vi "AssembleVelocityStats.vi"(7 "TitlePrefix":string, 10 "DataIn":T1) -> (1 "Plug in titles":string[](array[string]), 3 "StatsArray":dbl[](array[numeric]))   [LabVIEW 2020]
uses:
  <vilib>/Analysis/baseanly.llb/Unimode.vi
  <vilib>/Analysis/NI_AALBase.lvlib
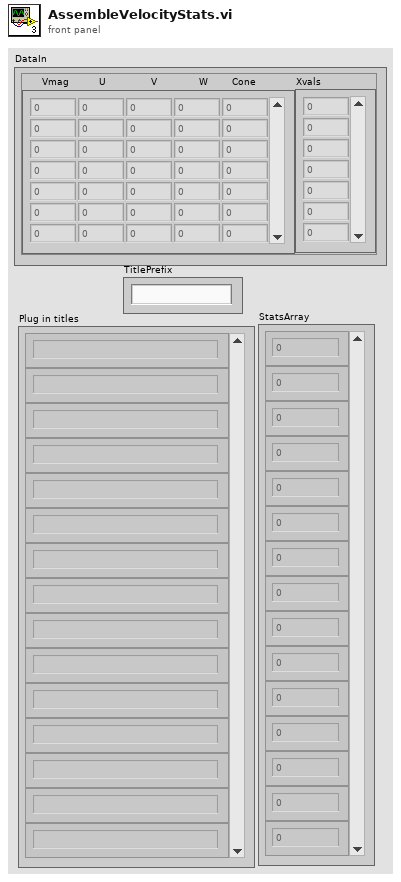
[diagram p1: front panel]
types:
  T1 = cluster{"   Vmag          U               V              W        Cone":dbl[][], "Xvals":i32[]}
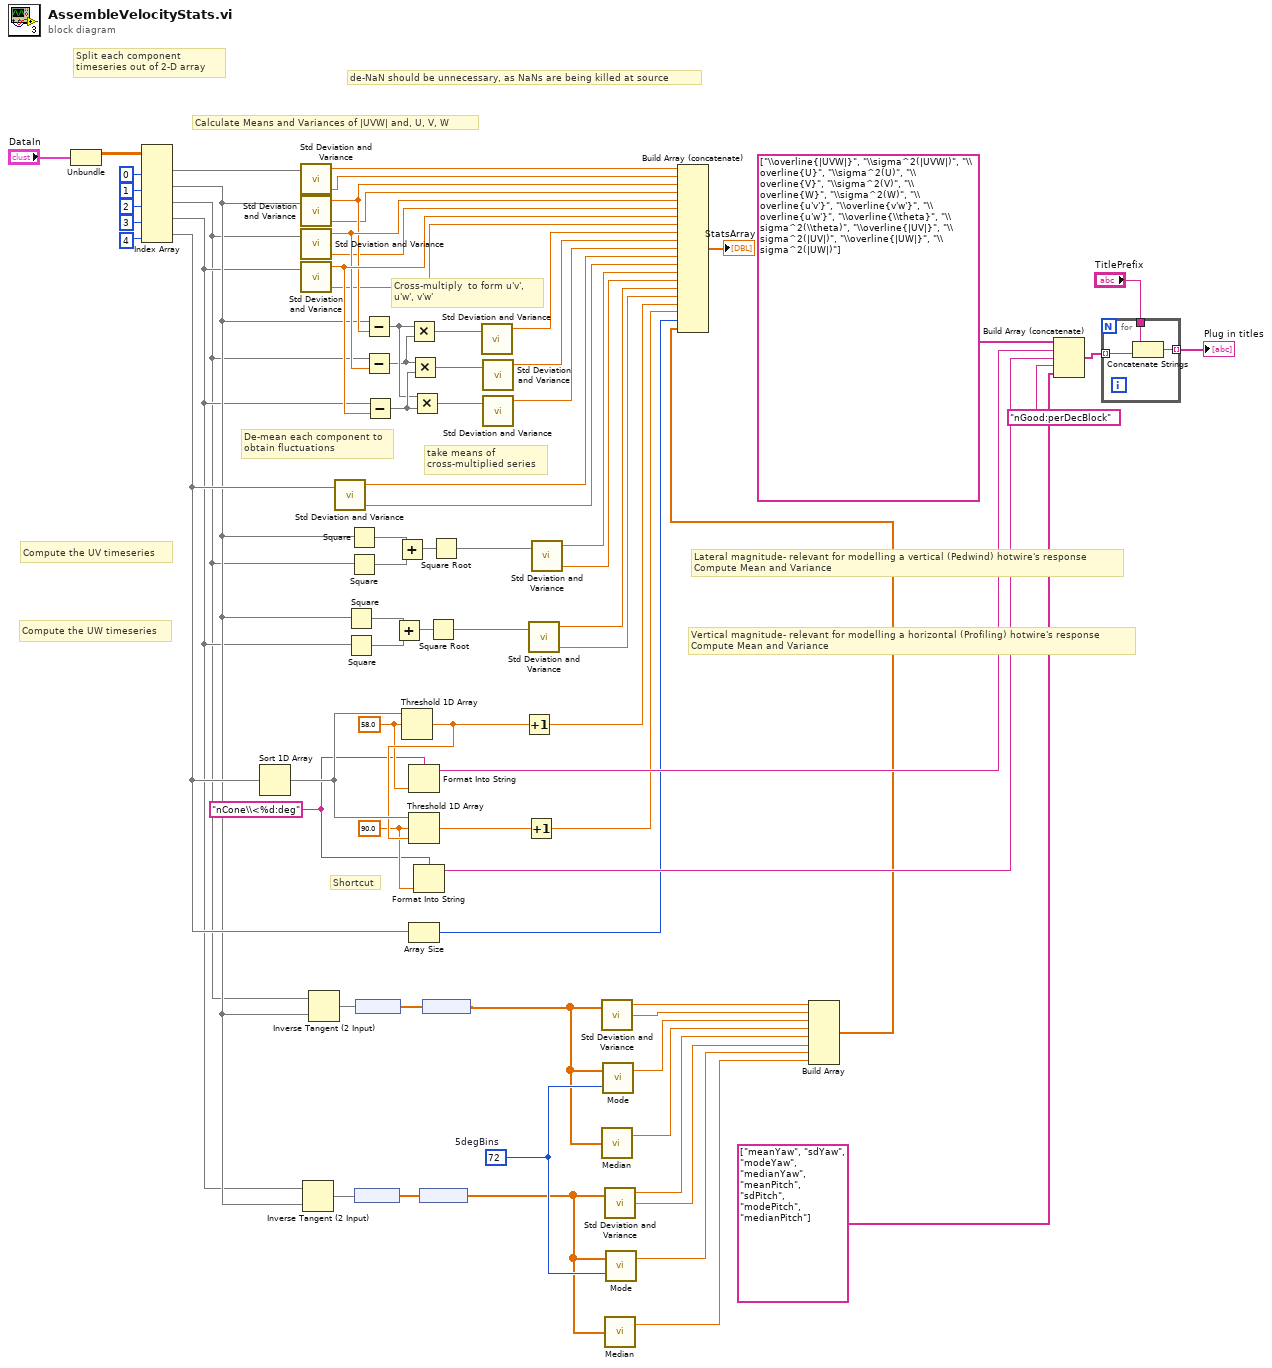
[diagram p0: block diagram]
diagram:
  w13 = 72  # 5degBins
  w31 = "nCone\\<%d:deg" ("format string")
  w32 = 90.0 ("threshold y")
  w33 = 58.0 ("threshold y")
  # "Split each component timeseries out of 2-D array"
  # "Compute the UW timeseries"
  # "Compute the UV timeseries"
  # "take means of cross-multiplied series"
  # "Cross-multiply  to form u'v', u'w', v'w'"
  # "De-mean each component to obtain fluctuations"
  # "Calculate Means and Variances of |UVW| and, U, V, W"
  # "Shortcut"
  # "de-NaN should be unnecessary, as NaNs are being killed at source"
  # "Vertical magnitude- relevant for modelling a horizontal (Profiling) hotwire's response\nCompute Mean and Variance"
  # "Lateral magnitude- relevant for modelling a vertical (Pedwind) hotwire's response\nCompute Mean and Variance"
  n1 = Unbundle("DataIn") -> ("Vmag          U               V              W        Cone"=w26:dbl[][])  [unwired: 1 out]
  n2 = Index Array(array=w26, index (col) #1=0 ("disabled index (col)"), index (col) #2=1 ("index (col)"), index (col) #3=2 ("index (col)"), index (col) #4=3 ("index (col)"), index (col) #5=4 ("index (col)")) -> (element #1=w25:dbl[], element #2=w20:dbl[], element #3=w18:dbl[], element #4=w19:dbl[], element #5=w37:dbl[])  [unwired: 5 in]
  n3 = Sort 1D Array(array=w37) -> (sorted array=w36:dbl[])
  n4 = call <vilib>:"Std Deviation and Variance.vi"("X"=w25) -> ("mean"=w65:dbl, "variance"=w60:dbl)  [unwired: 1 in, 1 out]
  n5 = call <vilib>:"Std Deviation and Variance.vi"("X"=w20) -> ("mean"=w66:dbl, "variance"=w61:dbl)  [unwired: 1 in, 1 out]
  n6 = call <vilib>:"Std Deviation and Variance.vi"("X"=w18) -> ("mean"=w67:dbl, "variance"=w62:dbl)  [unwired: 1 in, 1 out]
  n7 = call <vilib>:"Std Deviation and Variance.vi"("X"=w19) -> ("mean"=w68:dbl, "variance"=w63:dbl)  [unwired: 1 in, 1 out]
  n8 = Inverse Tangent (2 Input)(1:w20, 2:w19) -> (0:w15:dbl[])
  n9 = Inverse Tangent (2 Input)(1:w20, 2:w18) -> (0:w14:dbl[])
  n10 = call <vilib>:"Std Deviation and Variance.vi"("X"=w37) -> ("mean"=w76:dbl, "variance"=w77:dbl)  [unwired: 1 in, 1 out]
  n11 = Square(x=w20) -> (x^2=w40:dbl[])
  n12 = Square(x=w19) -> (x^2=w41:dbl[])
  n13 = Square(x=w20) -> (x^2=w49:dbl[])
  n14 = Square(x=w18) -> (x^2=w48:dbl[])
  n15 = node(w15) -> (w16:dbl[unit][])
  n16 = node(w14) -> (w17:dbl[unit][])
  n17 = Subtract(x=w20, y=w66) -> (x-y=w70:dbl[])
  n18 = Subtract(x=w18, y=w67) -> (x-y=w69:dbl[])
  n19 = Subtract(x=w19, y=w68) -> (x-y=w71:dbl[])
  n20 = Add(x=w40, y=w41) -> (x+y=w42:dbl[])
  n21 = Add(x=w49, y=w48) -> (x+y=w47:dbl[])
  n22 = Threshold 1D Array(2:w33, 3:w36) -> (0:w35:dbl)  [unwired: 1 in]
  n23 = Multiply(x=w70, y=w69) -> (x*y=w52:dbl[])
  n24 = Format Into String(format string=w31, w33) -> (resulting string=w29:string)  [unwired: 2 in, 1 out]
  n25 = Threshold 1D Array(1:w35, 2:w32, 3:w36) -> (0:w34:dbl)
  n26 = Array Size(array=w37) -> (size(s)=w23:i32)
  n27 = Multiply(x=w69, y=w71) -> (x*y=w51:dbl[])
  n28 = Multiply(x=w70, y=w71) -> (x*y=w50:dbl[])
  n29 = Format Into String(format string=w31, w32) -> (resulting string=w28:string)  [unwired: 2 in, 1 out]
  n30 = node(w16) -> (w11:dbl[])
  n31 = node(w17) -> (w12:dbl[])
  n32 = Square Root(x=w42) -> (sqrt(x)=w43:dbl[])
  n33 = Square Root(x=w47) -> (sqrt(x)=w46:dbl[])
  n34 = call <vilib>:"Std Deviation and Variance.vi"("X"=w52) -> ("mean"=w72:dbl)  [unwired: 1 in, 2 out]
  n35 = call <vilib>:"Std Deviation and Variance.vi"("X"=w51) -> ("mean"=w73:dbl)  [unwired: 1 in, 2 out]
  n36 = call <vilib>:"Std Deviation and Variance.vi"("X"=w50) -> ("mean"=w74:dbl)  [unwired: 1 in, 2 out]
  n37 = Increment(x=w35) -> (x+1=w22:dbl)
  n38 = Increment(x=w34) -> (x+1=w21:dbl)
  n39 = call <vilib>:"Std Deviation and Variance.vi"("X"=w43) -> ("mean"=w39:dbl, "variance"=w38:dbl)  [unwired: 1 in, 1 out]
  n40 = call <vilib>:"Std Deviation and Variance.vi"("X"=w46) -> ("mean"=w45:dbl, "variance"=w44:dbl)  [unwired: 1 in, 1 out]
  n41 = call <vilib>:"Std Deviation and Variance.vi"("X"=w12) -> ("mean"=w10:dbl, "standard deviation"=w9:dbl)  [unwired: 1 in, 1 out]
  n42 = call <vilib>:"Median.vi"("X"=w12) -> ("median"=w7:dbl)  [unwired: 1 out]
  n43 = call-poly <vilib>:"Mode.vi"("intervals"=w13, "X"=w12) -> ("mode"=w8:dbl)  [unwired: 1 out]
  n44 = call <vilib>:"Std Deviation and Variance.vi"("X"=w11) -> ("mean"=w6:dbl, "standard deviation"=w5:dbl)  [unwired: 1 in, 1 out]
  n45 = call <vilib>:"Median.vi"("X"=w11) -> ("median"=w3:dbl)  [unwired: 1 out]
  n46 = call-poly <vilib>:"Mode.vi"("intervals"=w13, "X"=w11) -> ("mode"=w4:dbl)  [unwired: 1 out]
  n47 = Build Array(w10, w9, w8, w7, w6, w5, w4, w3) -> (w2:dbl[])
  n48 = Build Array (concatenate)(w65, w60, w66, w61, w67, w62, w68, w63, w72, w73, w74, w76, w77, w45, w44, w39, w38, w22, w21, w23, w2) -> (→"StatsArray":dbl[])
  n49 = Build Array (concatenate)(string[] ["\\overline{|UVW|}", "\\sigma^2(|UVW|)", "\\overline{U}", "\\sigma^2(U)", "\\overline{V}", "\\sigma^2(V)", "\\overline{W}", "\\sigma^2(W)", "\\overline{u'v'}", "\\overline{v'w'}", "\\overline{u'w'}", "\\overline{\\theta}", "\\sigma^2(\\theta)", "\\overline{|UV|}", "\\sigma^2(|UV|)", "\\overline{|UW|}", "\\sigma^2(|UW|)"] ("Plug in titles"), w29, w28, "nGood:perDecBlock", string[] ["meanYaw", "sdYaw", "modeYaw", "medianYaw", "meanPitch", "sdPitch", "modePitch", "medianPitch"]) -> (w30:string[])
  n50 = for {
    tunnel: w30 -> [w80] mode=indexing
    tunnel: "TitlePrefix" -> [w79]
    tunnel: [w78] -> w53 mode=indexing
    n51 = Concatenate Strings(w79, w80) -> (w78:string)
  }
  "Plug in titles" <- w53
